vi "Dialog_control_DC_power_BM.vi"(0 "Enable":bool=TRUE, 5 "error in (no error)":errorcluster) -> (14 "Current":string, 15 "Voltage":string, 16 "Channel":string, 17 "Power (T = on, F = Off)":bool, 18 "OK":bool, 19 "error out":errorcluster)   [LabVIEW 2021]
doc: "Displays a standard dialog box that prompts users to enter information, such as a user name and password.\n--------------------\n\nThis Express VI is configured as follows:\n\nMessage to Display to the User:Turn on/off DC power supply to electrochemical cell.\nThe inputs are: \nCheckbox: Power (T = on, F = Off)\nText Entry Box: Channel\nText Entry Box: Voltage\nText Entry Box: Current"
panel:
  in  "Current":string="1.0"
  in  "Voltage":string="4.0"
  in  "Channel":string="1"
  in  "Power (T = on, F = Off)":bool
  out "String":string="Turn on/off DC power supply to electrochemical cell."
  in  "Cancel":bool
  in  "OK2":bool
  in  "OK1":bool
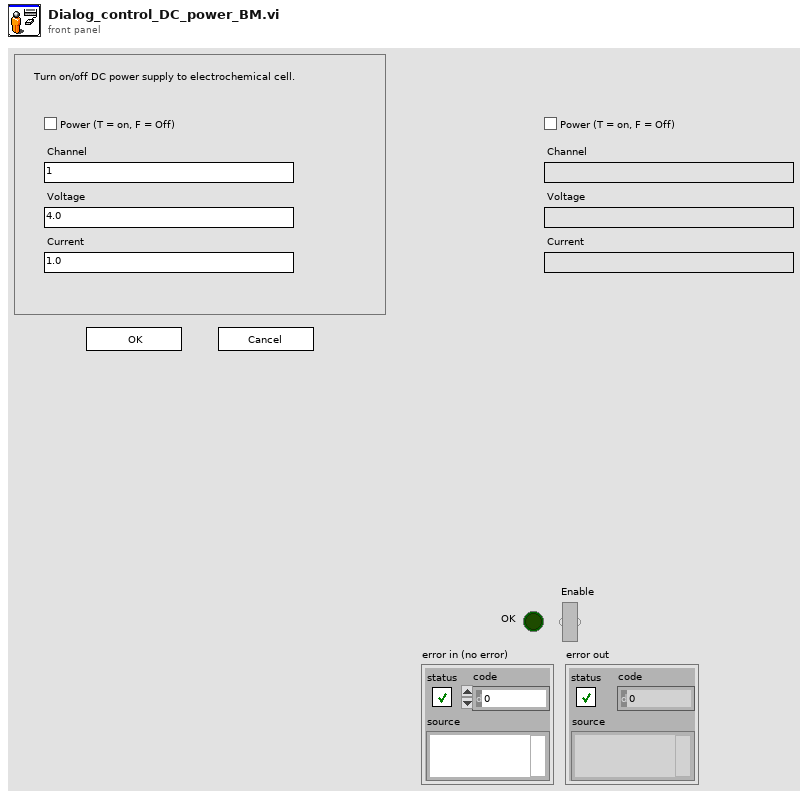
[diagram p1: front panel]
types:
  T1 = cluster{"Input Name":string, "Input Data Type":i32}[]
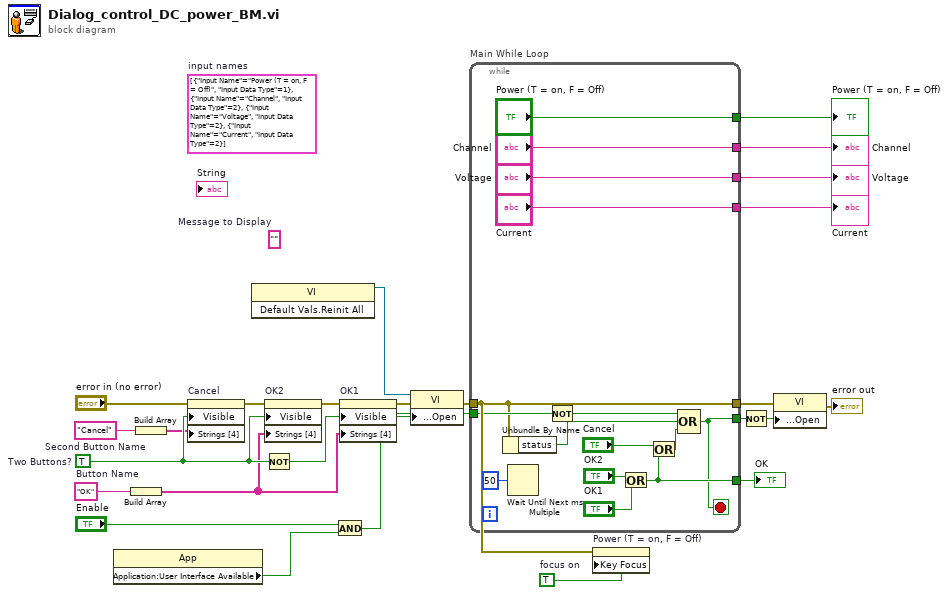
[diagram p0: block diagram]
diagram:
  w4 = TRUE  # focus on
  (unwired) T1 [{"Input Name"="Power (T = on, F = Off)", "Input Data Type"=1}, {"Input Name"="Channel", "Input Data Type"=2}, {"Input Name"="Voltage", "Input Data Type"=2}, {"Input Name"="Current", "Input Data Type"=2}]  # input names
  w17 = "Cancel"  # Second Button Name
  w15 = "OK"  # Button Name
  (unwired) ""  # Message to Display
  w25 = TRUE  # Two Buttons?
  n1 = property class="App"() -> ("Application:User Interface Available"=w7:bool)  [unwired: 2 in, 2 out]
  n2 = Build Array(w15) -> (w16:string[])
  n3 = Build Array(w17) -> (w18:string[])
  n4 = property on="Cancel" class="Bool"(error in="error in (no error)", "Visible"=w25, "Strings [4]"=w18) -> (error out=w22:errorcluster)  [unwired: 1 in, 1 out]
  n5 = invoke class="VI" method="Default Vals.Reinit All"() -> (reference out=w6:refnum<vi>)  [unwired: 3 in, 2 out]
  n6 = Not(x=w25) -> (.not. x?=w23:bool)
  n7 = property on="OK2" class="Bool"(error in=w22, "Visible"=w25, "Strings [4]"=w16) -> (error out=w21:errorcluster)  [unwired: 1 in, 1 out]
  n8 = And(x="Enable", y=w7) -> (x .and. y?=w8:bool)
  n9 = property on="OK1" class="Bool"(error in=w21, "Visible"=w23, "Strings [4]"=w16) -> (error out=w14:errorcluster)  [unwired: 1 in, 1 out]
  n10 = property class="VI"(reference=w6, error in=w14, "Front Panel Window:Open"=w8) -> (error out=w13:errorcluster)  [unwired: 1 out]
  n11 = while "Main While Loop" {
    tunnel: [w37] -> w24
    tunnel: w8 -> [w35]
    tunnel: [w33] -> w19
    tunnel: w13 -> [w32]
    tunnel: [w32] -> w11
    tunnel: ["Power (T = on, F = Off)"] -> w5
    tunnel: ["Channel"] -> w3
    tunnel: ["Voltage"] -> w2
    tunnel: ["Current"] -> w1
    stop <- w33 stop-if-true
    n12 = Unbundle By Name(w32) -> ("status"=w30:bool)
    n13 = Wait Until Next ms Multiple(millisecond multiple=u32 50) -> ()  [unwired: 1 out]
    n14 = Not(x=w35) -> (.not. x?=w34:bool)
    n15 = Or(x="OK2", y="OK1") -> (x .or. y?=w37:bool)
    n16 = Or(x="Cancel", y=w37) -> (x .or. y?=w31:bool)
    n17 = Compound Arithmetic op=OR(w34, w30, w31) -> (w33:bool)
  }
  "OK" <- w24
  "Power (T = on, F = Off)" <- w5
  "Channel" <- w3
  "Voltage" <- w2
  "Current" <- w1
  n18 = property on="Power (T = on, F = Off)" class="Bool (strict)"(error in=w13, "Key Focus"=w4) -> ()  [unwired: 1 in, 2 out]
  n19 = Not(x=w19) -> (.not. x?=w20:bool)
  n20 = property class="VI"(error in=w11, "Front Panel Window:Open"=w20) -> (error out=→"error out":errorcluster)  [unwired: 1 in, 1 out]
